vi "ANDO_IRTF_tracedownload_2011 version.vi"() -> ()   [LabVIEW 2011]
uses:
  <instrlib>/Generators/filename generator (time).vi
  <vilib>/Utility/file.llb/Write To Spreadsheet File (DBL).vi
  <instrlib>/Filename Generator.lvlib
panel:
  in  "filename root":string="1560nm" caption="filename root (none)"
  in  "seconds to wait":u32=10
  in  "stop":bool
  out "XY Graph":cluster{"Wavelength":sgl[], "Level":sgl[]}(graph)
  in  "export path":path=path "C:/Users/VGroup/Desktop/data/20140617"
  in  "Save data?":bool=TRUE
  out "Error Out":errorcluster
  in  "Error In":errorcluster
  in  "Trace (0:A)":enum16{"A", "B", "C"}(ring)
  in  "VISA session":refnum<visa-resource-name>="GPIB0::1::INSTR"
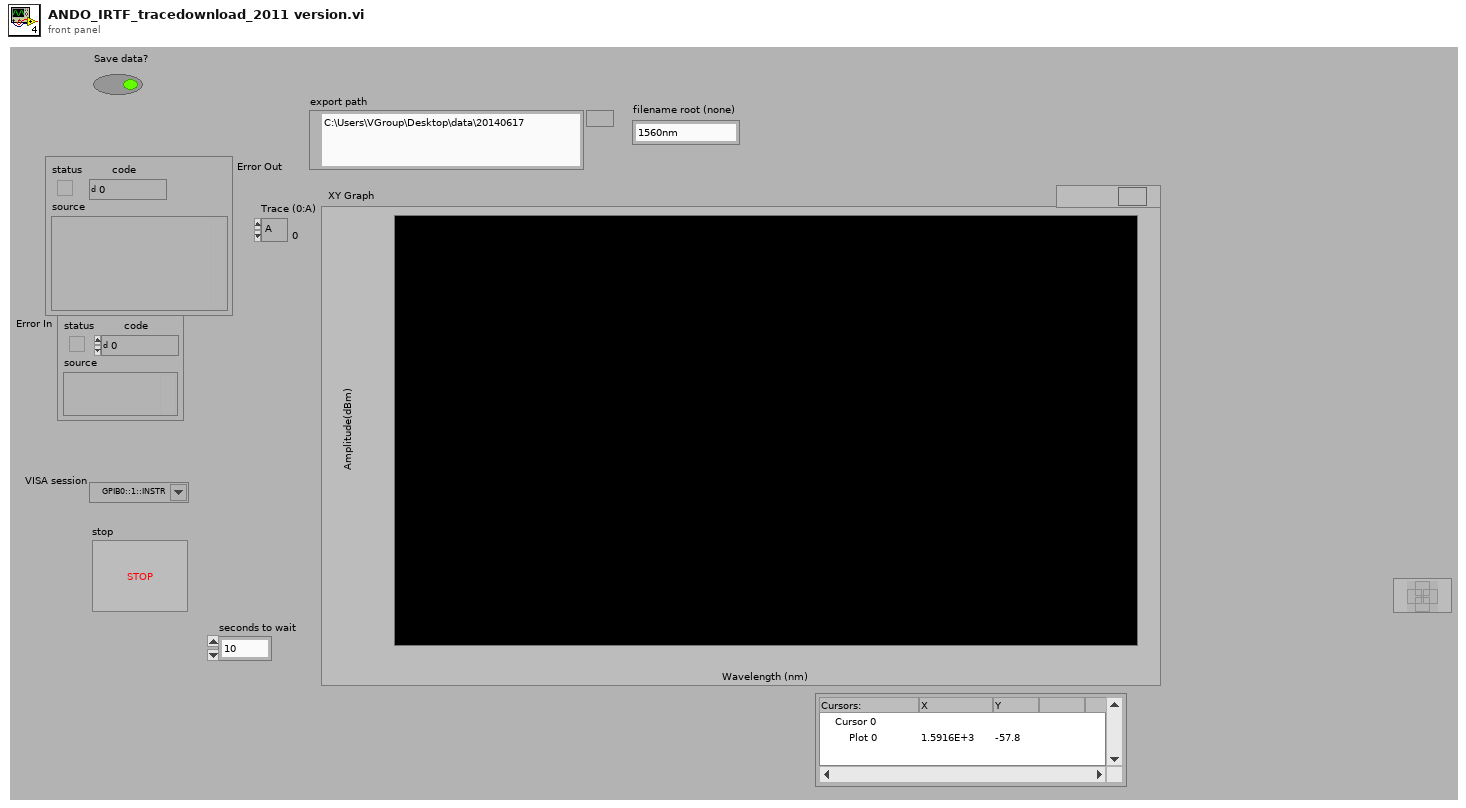
[diagram p1: front panel]
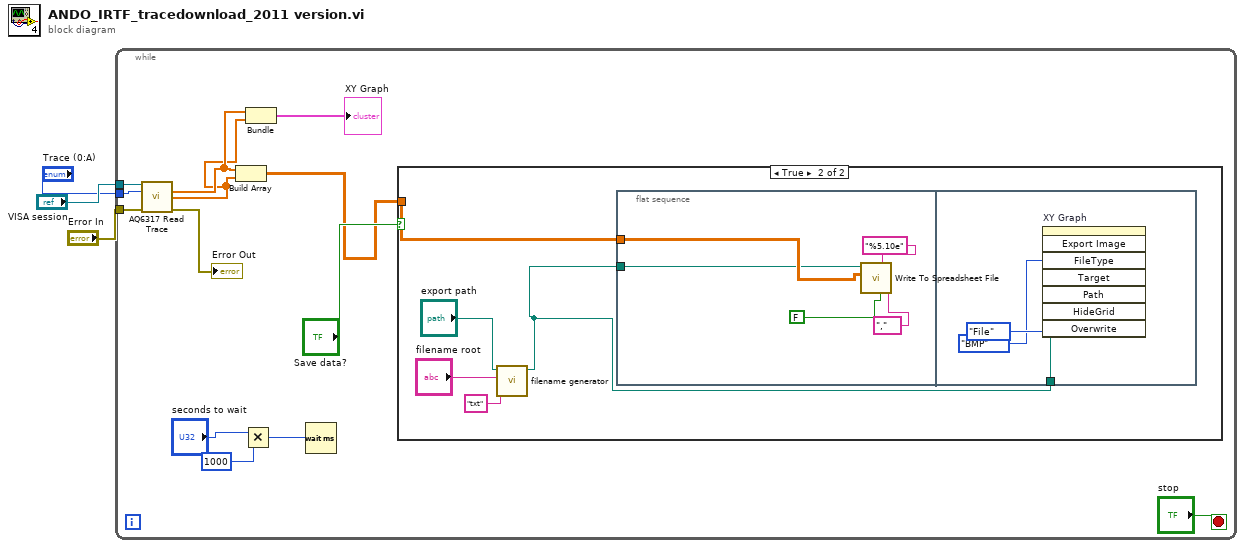
[diagram p0: block diagram]
diagram:
  n1 = while {
    tunnel: "VISA session" -> [w16]
    tunnel: "Trace (0:A)" -> [w15]
    tunnel: "Error In" -> [w14]
    stop <- "stop" stop-if-true
    n2 = call <instrlib>:"AQ6317 Read Trace.vi"("VISA session"=w16, "Trace (0:A)"=w15, "Error In"=w14) -> ("Wavelength"=w10:sgl[], "Level"=w9:sgl[], "Error Out"=→"Error Out":errorcluster)  [unwired: 7 in, 3 out]
    n3 = Build Array(w10, w9) -> (w11:sgl[][])
    n4 = Multiply(x="seconds to wait", y=u32 1000) -> (x*y=w4:u32)
    n5 = Bundle("Wavelength"=w10, "Level"=w9) -> (→"XY Graph":cluster{"Wavelength":sgl[], "Level":sgl[]})  [unwired: 1 in]
    n6 = Wait (ms)(milliseconds to wait=w4) -> ()  [unwired: 1 out]
    n7 = case shown="True" "Save data?" {
      tunnel: w11 -> [_ w21]
      frame False {
      }
      frame True {
        n8 = call-poly <instrlib>:"filename generator.vi"("extension"="txt", "filename root"="filename root", "root folder"="export path") -> ("filename"=w19:path)  [unwired: 7 in, 1 out]
        n9 = flat-sequence {
          tunnel: w21 -> [w26]
          tunnel: w19 -> [w22]
          tunnel: w19 -> [w27]
          frame #0 {
            n10 = call-poly <vilib>:"Write To Spreadsheet File.vi"("delimiter (\\t)"="," ("delimiter (Tab)"), "transpose? (no:F)"=FALSE, "format (%.3f)"="%5.10e", "2D data"=w26, "file path (dialog if empty)"=w22) -> ()  [unwired: 3 in, 1 out]
          }
          frame #1 {
            n11 = invoke on="XY Graph" class="XYGraph (strict)" method="Export Image"("FileType"=enum32{"BMP", "EPS", "EMF", "PICT"}."BMP" ("File Type"), "Target"=enum32{"File", "Clipboard"}."File", "Path"=w27) -> ()  [unwired: 5 in, 8 out]
          }
        }
      }
    }
  }
